vi "AdaptToInputs.vi"(0 "XRef":T16, 1 "Term Types":T13, 2 "State In":T1) -> (14 "Reply":T11, 15 "Fatal Error Out":T10, 16 "State Out":T1)   [LabVIEW 2020, in "FlexBlock.xnode"]
uses:
  FlexBlock.xnode
  <vilib>/XNodeSupport/XNodeXNodeRef.ctl
  <vilib>/XNodeSupport/XNodeTermTypeIDPairs.ctl
  <vilib>/XNodeSupport/XNodeTermTypeIDPair.ctl
  <vilib>/XNodeSupport/XNodeType.ctl
  <vilib>/XNodeSupport/XNodeString.ctl
  State.ctl
  FlexBlocks/Type Descriptor.ctl
  FlexBlocks/Terminal Direction.ctl
  FlexBlocks/Value Mode.ctl
  FlexBlocks/Terminal State.ctl
  FlexBlocks/Special Terminal.ctl
  FlexBlocks/Errors.ctl
  <vilib>/picture/picture.llb/imagedata.ctl
  FlexBlocks/Calculated Sizes.ctl
  <vilib>/XNodeSupport/XNodeStringArray.ctl
  <vilib>/XNodeSupport/XNodeErrorCluster.ctl
  <vilib>/XNodeSupport/NI_XNodeSupport.lvlib
  FlexBlocks/FlexBlocks.lvlib
  <vilib>/Utility/Data Type/NI_Data Type.lvlib
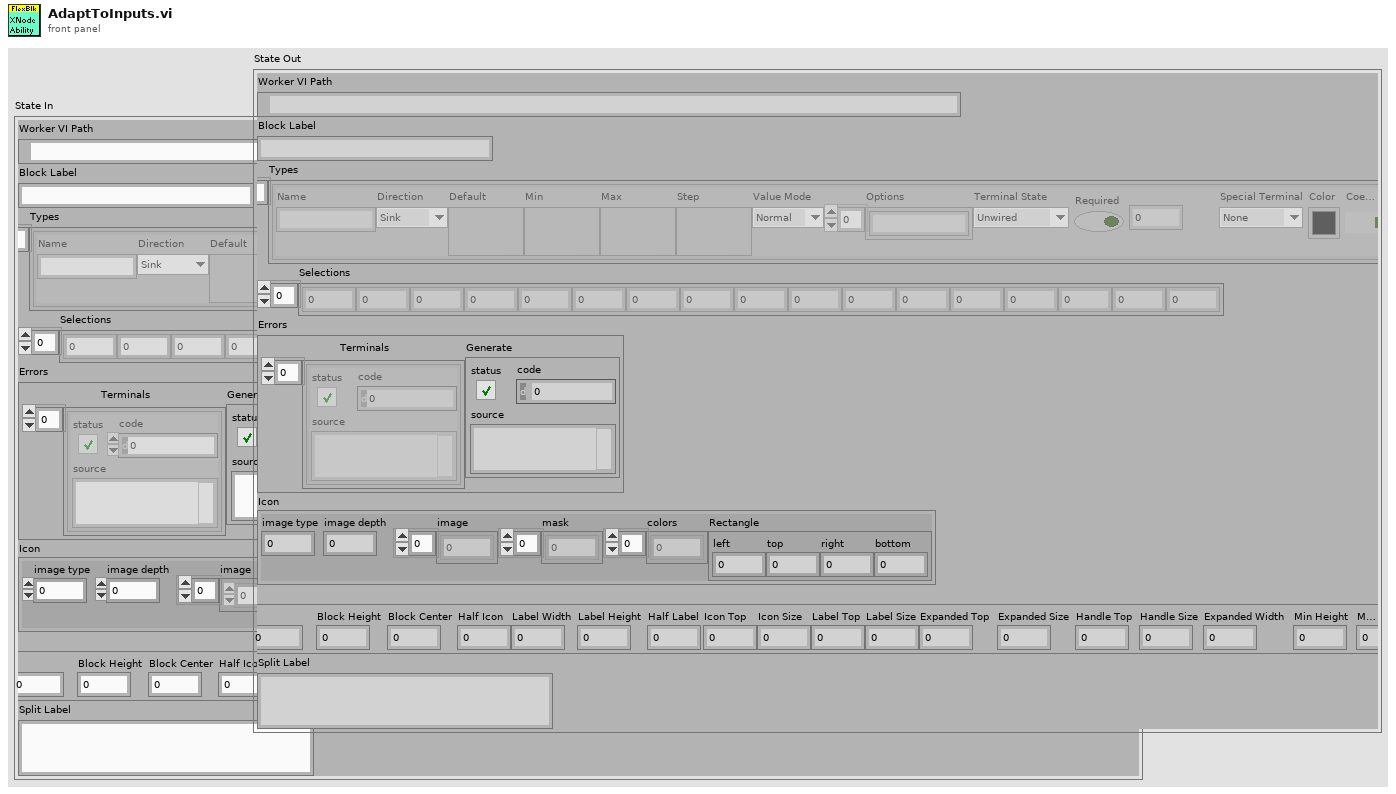
[diagram p1: front panel]
types:
  T1 = typedef "FlexBlock.xnode/State.ctl" = cluster{"Worker VI Path":path, "Block Label":string, "Types":T2[], "Selections":i32[], "Errors":T7, "Icon":T8, "Calcd Sizes":T9, "Split Label":string}
  T2 = typedef "FlexBlocks.lvlib/Type Descriptor.ctl" = cluster{"Name":string, "Direction":T3, "Default":variant, "Min":variant, "Max":variant, "Step":variant, "Value Mode":T4, "Options":string[], "Terminal State":T5, "Required":bool, "Connpane Index":i32, "Special Terminal":T6, "Color":u32, "Coerced":bool}
  T3 = typedef "FlexBlocks.lvlib/Terminal Direction.ctl" = enum16{"Sink", "Source"}
  T4 = typedef "FlexBlocks.lvlib/Value Mode.ctl" = enum16{"Normal", "Range", "Select"}
  T5 = typedef "FlexBlocks.lvlib/Terminal State.ctl" = enum16{"Unwired", "BadType", "BadRef", "Channel", "Value", "Control Ref"}
  T6 = typedef "FlexBlocks.lvlib/Special Terminal.ctl" = enum16{"None", "Action", "Init", "Tag", "State in", "State out", "Error"}
  T7 = typedef "FlexBlocks.lvlib/Errors.ctl" = cluster{"Terminals":errorcluster[], "Generate":errorcluster}
  T8 = typedef "imagedata.ctl" = cluster{"image type":i32, "image depth":i32, "image":u8[], "mask":u8[], "colors":u32[], "Rectangle":cluster{"left":i16, "top":i16, "right":i16, "bottom":i16}}
  T9 = typedef "FlexBlocks.lvlib/Calculated Sizes.ctl" = cluster{"Text Width":i32, "Text Height":i32, "Half Text":i32, "Block Width":i32, "Block Height":i32, "Block Center":i32, "Half Icon":i32, "Label Width":i32, "Label Height":i32, "Half Label":i32, "Icon Top":i32, "Icon Size":i32, "Label Top":i32, "Label Size":i32, "Expanded Top":i32, "Expanded Size":i32, "Handle Top":i32, "Handle Size":i32, "Expanded Width":i32, "Min Height":i32, "Max Height":i32}
  T10 = typedef "NI_XNodeSupport.lvlib/XNodeErrorCluster.ctl" = errorcluster
  T11 = typedef "NI_XNodeSupport.lvlib/XNodeStringArray.ctl" = T12[]
  T12 = typedef "NI_XNodeSupport.lvlib/XNodeString.ctl" = string
  T13 = typedef "NI_XNodeSupport.lvlib/XNodeTermTypeIDPairs.ctl" = T14[]
  T14 = typedef "NI_XNodeSupport.lvlib/XNodeTermTypeIDPair.ctl" = cluster{"Type":T15, "Id":T12}
  T15 = typedef "NI_XNodeSupport.lvlib/XNodeType.ctl" = variant
  T16 = typedef "NI_XNodeSupport.lvlib/XNodeXNodeRef.ctl" = refnum<vi>
  T17 = typedef "NI_Data Type.lvlib/Data Type.ctl" = enum8{"Invalid Type", "Void", "I8", "I16", "I32", "I64", "U8", "U16", "U32", "U64", "Single Float", "Double Float", "Extended Float", "Single Complex", "Double Complex", "Extended Complex", "Enum U8", "Enum U16", "Enum U32", "Enum U64", "Single Float With Unit", "Double Float With Unit", "Extended Float With Unit", "Single Complex with Unit", "Double Complex with Unit", "Extended Complex with Unit", "Boolean", "String", "Path", "Picture", "Tag", "Array", "Cluster", "Variant", "LV Variant", "Waveform", "Timestamp", "Digital Waveform", "Digital Data", "ExpressData", "Refnum", "External Data", "VI", "Poly VI", "LabVIEW Class Instance", "Fixed Point", "Set Collection", "Map Collection"}
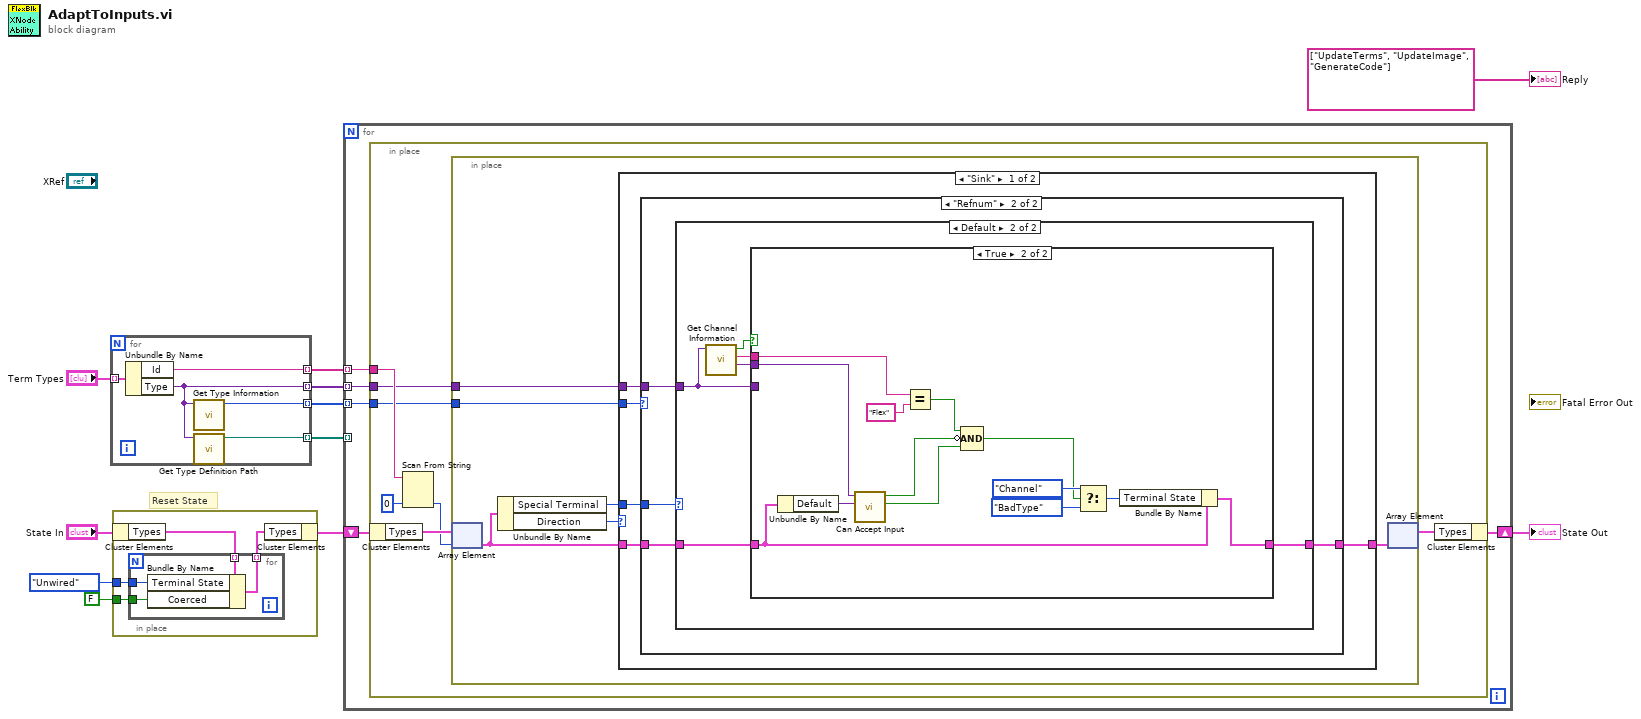
[diagram p0: block diagram]
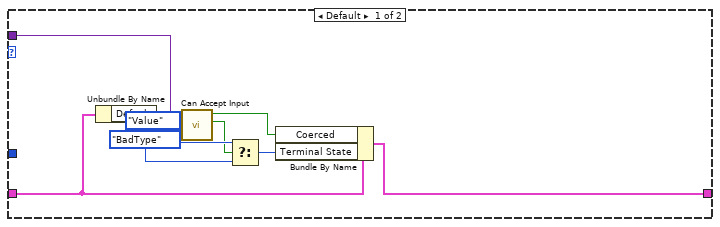
[diagram p2: hidden frame]
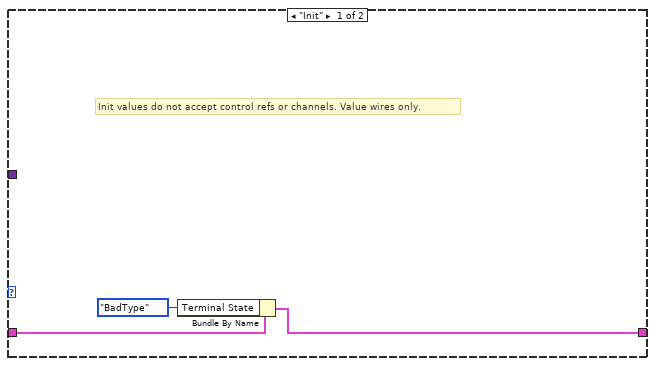
[diagram p3: hidden frame]
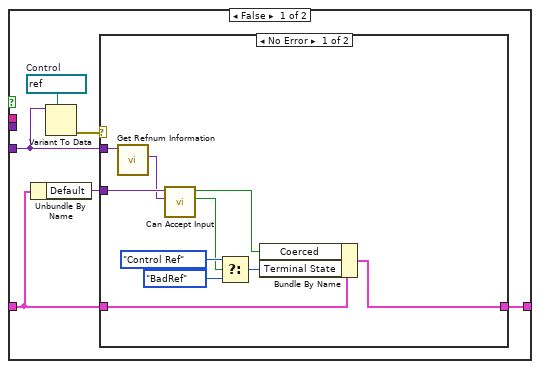
[diagram p4: hidden frame]
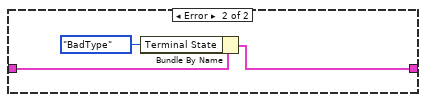
[diagram p5: hidden frame]
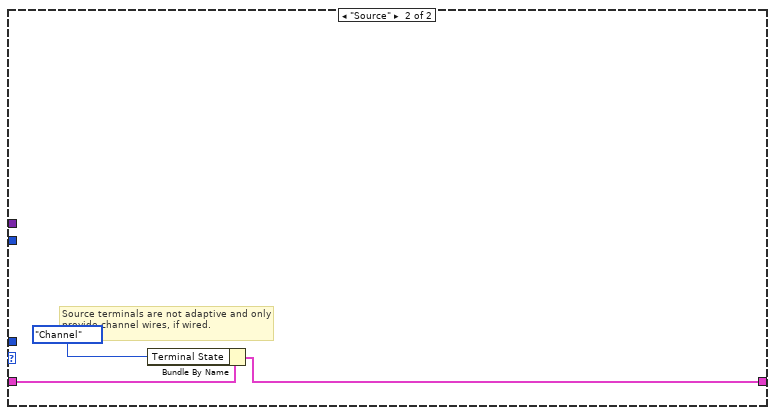
[diagram p6: hidden frame]
diagram:
  # "Reset State"
  n1 = for {
    tunnel: "Term Types" -> [w16] mode=indexing
    tunnel: [w15] -> w6 mode=indexing
    tunnel: [w14] -> w5 mode=indexing
    tunnel: [w13] -> w4 mode=indexing
    tunnel: [w12] -> w1 mode=indexing
    n2 = Unbundle By Name(w16) -> ("Id"=w14:T12, "Type"=w13:T15)
    n3 = call <vilib>:"Get Type Information.vi"("variant"=w13) -> ("type"=w15:T17)  [unwired: 6 in, 4 out]
    n4 = call <vilib>:"Get Type Definition Path.vi"("variant"=w13) -> ("type definition path"=w12:path)  [unwired: 9 in, 1 out]
  }
  n5 = in-place {
    in-place-border: Terminal_State."Unwired" ("Terminal State") -> [w19]
    in-place-border: FALSE ("Coerced") -> [w17]
    n6 = in-place-cluster #1("State In") -> ("Types"=w20:T2[])
    n7 = for {
      tunnel: w20 -> [w24] mode=indexing
      tunnel: w19 -> [w23]
      tunnel: [w22] -> w18 mode=indexing
      tunnel: w17 -> [w21]
      n8 = Bundle By Name(cluster=w24, "Terminal State"=w23, "Coerced"=w21) -> (w22:T2)
    }
    n9 = in-place-cluster #1("Types"=w18) -> (w8:T1)
  }
  n10 = for {
    shift-right: [w27] -> w3
    shift-left: w8 -> [w28]
    tunnel: w6 -> [w25] mode=indexing
    tunnel: w5 -> [w29] mode=indexing
    tunnel: w4 -> [w26] mode=indexing
    tunnel: w1 -> [_] mode=indexing
    n11 = in-place {
      in-place-border: w29 -> [w36]
      in-place-border: w26 -> [w32]
      in-place-border: w25 -> [w31]
      n12 = in-place-cluster #2(w28) -> ("Types"=w34:T2[])
      n13 = Scan From String(input string=w36, default 1=0 ("default value 1")) -> (output 1=w33:i32)  [unwired: 3 in, 3 out]
      n14 = in-place {
        in-place-border: w32 -> [w40]
        in-place-border: w31 -> [w39]
        n15 = in-place-array #3(w34, w33) -> (w41:T2)
        n16 = Unbundle By Name(w41) -> ("Special Terminal"=w37:T6, "Direction"=w42:T3)
        n17 = case shown="\"Sink\"" w42 {
          tunnel: w41 -> [w47 w104]
          tunnel: w40 -> [w45 _]
          tunnel: w39 -> [w46 _]
          tunnel: [w44 w102] -> w38
          tunnel: w37 -> [w43 _]
          frame "Sink" {
            n18 = case shown="\"Refnum\"" w46 {
              tunnel: w47 -> [w53 w60]
              tunnel: w45 -> [w48 w58]
              tunnel: [w52 w59] -> w44
              tunnel: w43 -> [_ w57]
              frame Default {
                n19 = Unbundle By Name(w53) -> ("Default"=w50:variant)
                n20 = call "Can Accept Input.vi"("Input Type"=w48, "Dest Type"=w50) -> ("Can Accept?"=w49:bool, "Coercion Needed?"=w51:bool)  [unwired: 8 in]
                n21 = Select(t=Terminal_State."Value" ("Terminal State"), s=w49, f=Terminal_State."BadType" ("Terminal State")) -> (s? t:f=w54:T5)
                n22 = Bundle By Name(cluster=w53, "Coerced"=w51, "Terminal State"=w54) -> (w52:T2)
              }
              frame "Refnum" {
                n23 = case shown="Default" w57 {
                  tunnel: w60 -> [w63 w69]
                  tunnel: [w61 w66] -> w59
                  tunnel: w58 -> [_ w65]
                  frame "Init" {
                    # "Init values do not accept control refs or channels. Value wires only."
                    n24 = Bundle By Name(cluster=w63, "Terminal State"=Terminal_State."BadType") -> (w61:T2)
                  }
                  frame Default {
                    n25 = call <vilib>:"Get Channel Information.vi"("variant"=w65) -> ("element type"=w64:variant, "template name"=w67:string, "channel?"=w68:bool)  [unwired: 6 in, 2 out]
                    n26 = case shown="True" w68 {
                      tunnel: w69 -> [w71 w95]
                      tunnel: w67 -> [_ w101]
                      tunnel: [w73 w96] -> w66
                      tunnel: w65 -> [w72 _]
                      tunnel: w64 -> [_ w93]
                      frame False {
                        w75 = refnum<vi> refnum  # Control
                        n27 = Unbundle By Name(w71) -> ("Default"=w70:variant)
                        n28 = Variant To Data(type=w75, Variant=w72) -> (error out=w74:errorcluster)  [unwired: 1 in, 1 out]
                        n29 = case shown="No Error" w74 {
                          tunnel: w71 -> [w82 w88]
                          tunnel: [w80 w86] -> w73
                          tunnel: w72 -> [w85 _]
                          tunnel: w70 -> [w79 _]
                          frame No Error {
                            n30 = call <vilib>:"Get Refnum Information.vi"("variant"=w85) -> ("strict type"=w78:variant)  [unwired: 7 in, 3 out]
                            n31 = call "Can Accept Input.vi"("Input Type"=w78, "Dest Type"=w79) -> ("Can Accept?"=w77:bool, "Coercion Needed?"=w76:bool)  [unwired: 8 in]
                            n32 = Select(t=Terminal_State."Control Ref" ("Terminal State"), s=w77, f=Terminal_State."BadRef" ("Terminal State")) -> (s? t:f=w81:T5)
                            n33 = Bundle By Name(cluster=w82, "Coerced"=w76, "Terminal State"=w81) -> (w80:T2)
                          }
                          frame Error {
                            n34 = Bundle By Name(cluster=w88, "Terminal State"=Terminal_State."BadType") -> (w86:T2)
                          }
                        }
                      }
                      frame True {
                        n35 = Unbundle By Name(w95) -> ("Default"=w94:variant)
                        n36 = call "Can Accept Input.vi"("Input Type"=w94, "Dest Type"=w93) -> ("Can Accept?"=w90:bool, "Coercion Needed?"=w91:bool)  [unwired: 8 in]
                        n37 = Equal?(x=w101, y="Flex") -> (x = y?=w92:bool)
                        n38 = Compound Arithmetic op=AND(w92, invert w91, w90) -> (w89:bool)
                        n39 = Select(t=Terminal_State."Channel", s=w89, f=Terminal_State."BadType" ("Terminal State")) -> (s? t:f=w98:T5)
                        n40 = Bundle By Name(cluster=w95, "Terminal State"=w98) -> (w96:T2)
                      }
                    }
                  }
                }
              }
            }
          }
          frame "Source" {
            # "Source terminals are not adaptive and only provide channel wires, if wired."
            n41 = Bundle By Name(cluster=w104, "Terminal State"=Terminal_State."Channel") -> (w102:T2)
          }
        }
        n42 = in-place-array #3(w38) -> (w30:T2[])  [unwired: 1 out]
      }
      n43 = in-place-cluster #2("Types"=w30) -> (w27:T1)
    }
  }
  "State Out" <- w3
  "Reply" <- T11 ["UpdateTerms", "UpdateImage", "GenerateCode"] ("Reply")
